vi "Main-Maze_Solver.vi"() -> ()   [LabVIEW 2020]
uses:
  Controls/TileColor.ctl
  Controls/Scan_Data.ctl
panel:
  in  "ms Per Move":u32=500 step=100
  out "Maze":T1[][](array[typedef])
  in  "Maze Path":path=path "C:/Users/Luke Jarocki/Downloads/maze_2.jpg"
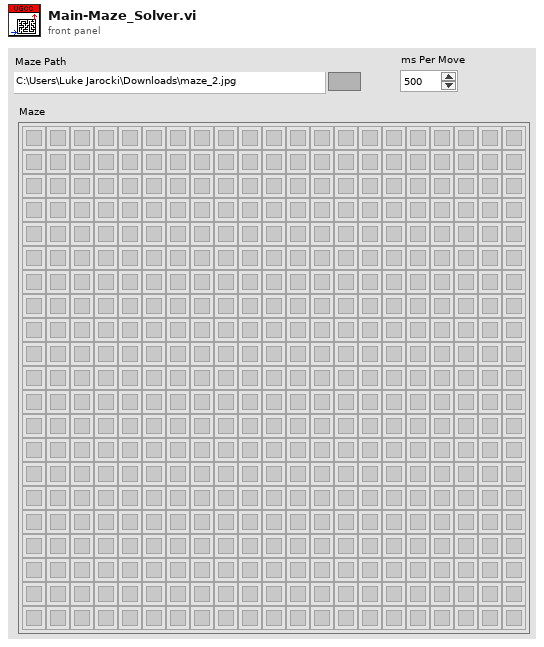
[diagram p1: front panel]
types:
  T1 = typedef "TileColor.ctl" = u16
  T2 = typedef "imagedata.ctl" = cluster{"image type":i32, "image depth":i32, "image":u8[], "mask":u8[], "colors":u32[], "Rectangle":cluster{"left":i16, "top":i16, "right":i16, "bottom":i16}}
  T3 = typedef "Scan_Data.ctl" = cluster{"X Dead Band":i32, "Y Dead Band":i32, "X Origin":i32, "Y Origin":i32, "Color Array":u32[][]}
  T4 = typedef "Scan_Values.ctl" = cluster{"Center Index":i32, "Scanned":bool, "Wall indices":i32[]}
  T5 = typedef "Parse-(X,Y).ctl" = cluster{"X":i32, "Y":i32, "Tile Color":T1}
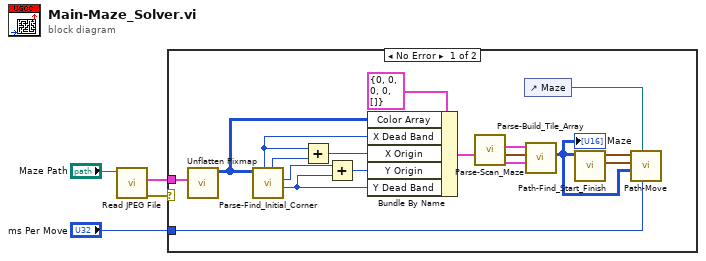
[diagram p0: block diagram]
diagram:
  n1 = call <vilib>:"Read JPEG File.vi"("path to JPEG file"="Maze Path") -> ("error out"=w1:errorcluster, "image data"=w4:T2)  [unwired: 8 in, 1 out]
  n2 = case shown="No Error" w1 {
    tunnel: w4 -> [w22 _]
    tunnel: "ms Per Move" -> [w6 _]
    frame No Error {
      n3 = call <vilib>:"Unflatten Pixmap.vi"("image data"=w22) -> ("24-bit pixmap"=w13:u32[][])  [unwired: 4 in, 6 out]
      n4 = call "Parse-Find_Initial_Corner.vi"("Color Array"=w13) -> ("Col Wall Thickness (px) (Y)"=w11:i32, "Origin Y"=w20:i32, "Origin X"=w19:i32, "Row Wall Thickness (px) (X)"=w15:i32)  [unwired: 5 in, 2 out]
      n5 = Add(x=w15, y=w19) -> (x+y=w14:i32)
      n6 = Add(x=w20, y=w11) -> (x+y=w12:i32)
      n7 = Bundle By Name(cluster=T3 {"X Dead Band"=0, "Y Dead Band"=0, "X Origin"=0, "Y Origin"=0, "Color Array"=[]} ("Scan"), "Color Array"=w13, "X Dead Band"=w15, "X Origin"=w14, "Y Origin"=w12, "Y Dead Band"=w11) -> (w10:T3)
      n8 = call "Parse-Scan_Maze.vi"("Scan Parameters"=w10) -> ("Rows"=w18:T4[], "Barrier Coords"=w21:T5[], "Columns"=w17:T4[])  [unwired: 8 in]
      n9 = control-ref of="Maze"() -> (w7:refnum<vi>)
      n10 = call "Parse-Build_Tile_Array.vi"("Rows"=w18, "Barrier Coords"=w21, "Columns"=w17) -> ("output array"=w5:T1[][])  [unwired: 8 in]
      "Maze" <- w5
      n11 = call "Path-Find_Start_Finish.vi"("Tile Array"=w5) -> ("Start"=w9:T5, "Finish"=w8:T5)  [unwired: 9 in]
      n12 = call "Path-Move.vi"("Move Time"=w6, "Maze Display Ref"=w7, "Tile Array"=w5, "Start"=w9, "Finish"=w8) -> ()  [unwired: 6 in, 1 out]
    }
    frame Error {
    }
  }
